vi "Begin.vi"(11 "Image Size":T1=enum."160x120") -> (0 "error out":errorcluster)   [LabVIEW 2012]
doc: "Called before other user functions, this VI is expected to open initial I/O refnums, load in file data, and do all program initialization. Notice that the <B>error out</B> terminal is simply used for data flow. Wiring it to other structures or subVIs ensures that this VI runs first."
uses:
  <vilib>/Rock Robotics/WPI/Camera/WPI_CameraImageSize.ctl
  <vilib>/Rock Robotics/WPI/Camera/WPI_CameraWhite Balance Values.ctl
  <vilib>/Rock Robotics/WPI/Camera/WPI_CameraExposure Values.ctl
  <vilib>/Rock Robotics/WPI/Camera/WPI_CameraFrameRate.ctl
  <vilib>/Rock Robotics/WPI/DriverStation/WPI_DriverStationRobotMode2.ctl
  <vilib>/Rock Robotics/WPI/Joystick/WPI_JoystickDeviceEnum.ctl
  <vilib>/Rock Robotics/SystemInterfaces/DIO/FPGA_DIOPWMChannel.ctl
  <vilib>/Rock Robotics/SystemInterfaces/Typedef/FPGA_TypedefDigitalModule.ctl
  <vilib>/Rock Robotics/SystemInterfaces/DIO/FPGA_DIORelayChannel.ctl
  <vilib>/Rock Robotics/WPI/Relay/WPI_RelayDirection.ctl
  <vilib>/Rock Robotics/WPI/AnalogChannel/WPI_AnalogChannelDevRef.ctl
  <vilib>/Rock Robotics/SystemInterfaces/Typedef/FPGA_TypedefAnalogModule.ctl
  <vilib>/Rock Robotics/SystemInterfaces/AI/FPGA_AIChannel.ctl
  <vilib>/Rock Robotics/SystemInterfaces/CounterEncoderSourceConvertion/FPGA_CounterEncoderSourceConvertionLVSourceType.ctl
  <vilib>/Rock Robotics/SystemInterfaces/DIO/FPGA_DIODigitalSourceChannel.ctl
  <vilib>/Rock Robotics/SystemInterfaces/AnalogTrigger/FPGA_AnalogTriggerIndex.ctl
  <vilib>/Rock Robotics/SystemInterfaces/AnalogTrigger/FPGA_AnalogTriggerOutType.ctl
  <vilib>/Rock Robotics/SystemInterfaces/AI/FPGA_AIGyroChannel.ctl
  <vilib>/Rock Robotics/SystemInterfaces/Typedef/FPGA_TypedefAnalogModuleForGyro.ctl
  <vilib>/Rock Robotics/SystemInterfaces/DIO/FPGA_DIOChannel.ctl
  <vilib>/Rock Robotics/WPI/Encoder/WPI_EncoderType.ctl
  Robot Global Data.vi
  <vilib>/Rock Robotics/WPI/RobotDrive/WPI_RobotDriveOpen2MotorWithJaguar.vi
  <vilib>/Rock Robotics/WPI/MotorControl/WPI_MotorControlOpen Victor.vi
  <vilib>/Rock Robotics/WPI/MotorControl/WPI_MotorControlOpen Jaguar.vi
  <vilib>/Rock Robotics/WPI/Counter/WPI_CounterOpen UpDown Mode.vi
  <vilib>/Rock Robotics/WPI/Counter/WPI_CounterDigitalInputToDigitalSource.vi
panel:
  out "error out 2":errorcluster
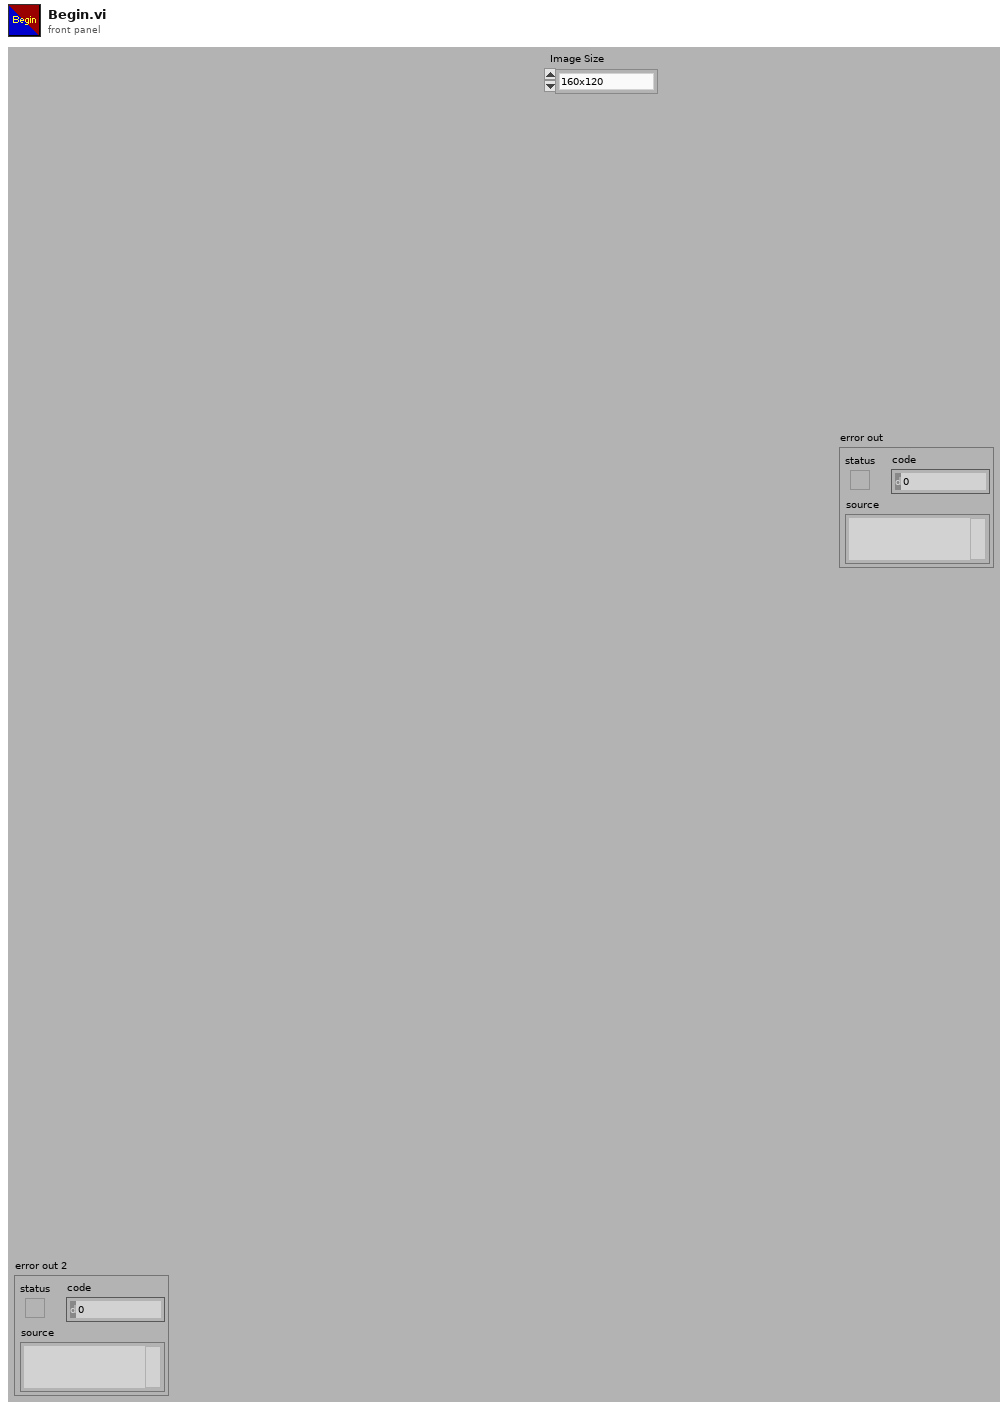
[diagram p1: front panel]
types:
  T1 = typedef "WPI_CameraImageSize.ctl" = enum16{"640x480", "320x240", "160x120"}
  T2 = typedef "WPI_RelayDirection.ctl" = enum16{"Both directions", "Forward only", "Reverse only"}
  T3 = typedef "FPGA_DIORelayChannel.ctl" = enum8{"Relay 1", "Relay 2", "Relay 3", "Relay 4", "Relay 5", "Relay 6", "Relay 7", "Relay 8", "Invalid"}
  T4 = typedef "FPGA_TypedefDigitalModule.ctl" = enum16{"Digital Module 1", "Digital Module 2"}
  T5 = typedef "FPGA_DIOPWMChannel.ctl" = enum8{"PWM 1", "PWM 2", "PWM 3", "PWM 4", "PWM 5", "PWM 6", "PWM 7", "PWM 8", "PWM 9", "PWM 10", "Invalid"}
  T6 = typedef "WPI_JoystickDeviceEnum.ctl" = enum16{"USB 1", "USB 2", "USB 3", "USB 4", "Kinect 1", "Kinect 2"}
  T7 = typedef "WPI_DriverStationRobotMode2.ctl" = enum16{"Autonomous Disabled", "Autonomous Enabled", "Teleop Disabled", "Teleop Enabled", "Timeout", "Finish", "Test Disabled", "Test Enabled"}
  T8 = typedef "WPI_CameraFrameRate.ctl" = u32
  T9 = typedef "WPI_CameraExposure Values.ctl" = enum16{"Auto", "Flicker-free 50 Hz", "Flicker-free 60 Hz", "Hold current"}
  T10 = typedef "WPI_CameraWhite Balance Values.ctl" = enum16{"Auto", "Fixed indoor", "Fixed outdoor 1", "Fixed outdoor 2", "Fixed fluorescent 1", "Fixed fluorescent 2", "Hold current"}
  T11 = enum16{"Rising Edge", "Falling Edge", "Raising & Falling Edge", "Disabled"}
  T12 = typedef "FPGA_CounterEncoderSourceConvertionLVSourceType.ctl" = cluster{"DevStatus":errorcluster, "AnalogTriggerMode?":bool, "DigitalMode":cluster{"Digital Module":T4, "DIO Channel":T13}, "AnalogTriggerMode":cluster{"AnalogTriggerIndex":T14, "OutputType":T15}}
  T13 = typedef "FPGA_DIODigitalSourceChannel.ctl" = enum8{"DIO 1", "DIO 2", "DIO 3", "DIO 4", "DIO 5", "DIO 6", "DIO 7", "DIO 8", "DIO 9", "DIO 10", "DIO 11", "DIO 12", "DIO 13", "DIO 14", "Disabled"}
  T14 = typedef "FPGA_AnalogTriggerIndex.ctl" = enum8{"Trig 0", "Trig 1", "Trig 2", "Trig 3", "Trig 4", "Trig 5", "Trig 6", "Trig 7", "Invalid"}
  T15 = typedef "FPGA_AnalogTriggerOutType.ctl" = enum16{"InWindow", "TriggerState", "Rising", "Falling"}
  T16 = typedef "WPI_AnalogChannelDevRef.ctl" = cluster{"DevStatus":errorcluster, "Analog Module":T17, "Analog Channel":T18}
  T17 = typedef "FPGA_TypedefAnalogModule.ctl" = enum16{"Analog Module 1", "Analog Module 2"}
  T18 = typedef "FPGA_AIChannel.ctl" = enum8{"AI 1", "AI 2", "AI 3", "AI 4", "AI 5", "AI 6", "AI 7", "AI 8", "Invalid"}
  T19 = typedef "FPGA_AnalogTriggerDevRef.ctl" = cluster{"DevStatus":errorcluster, "AnalogTriggerIndex":T14}
  T20 = typedef "WPI_CounterDevRef.ctl" = cluster{"DevStatus":errorcluster, "CntIndex":T21}
  T21 = typedef "FPGA_CounterCtrSystemIndex.ctl" = enum8{"Ctr 0", "Ctr 1", "Ctr 2", "Ctr 3", "Ctr 4", "Ctr 5", "Ctr 6", "Ctr 7", "Invalid"}
  T22 = typedef "WPI_MotorControlDeviceRef.ctl" = cluster{"DeviceStatus":errorcluster, "Type":enum16{"PWM", "CAN"}, "PWM":cluster{"Digital Module":T4, "PWM Channel":T5, "DeadBand":T23}, "CAN":cluster{"Device Number":u8, "Control Mode":T24, "Semaphore":T25, "Max Vout":dbl}, "Invert":bool, "TransformRef":T26, "InvTransformRef":T26}
  T23 = typedef "WPI_PWMDeadband.ctl" = cluster{"Name":string, "maxPositivePwm":i32, "minPositivePwm":i32, "centerPwm":i32, "maxNegativePwm":i32, "minNegativePwm":i32, "angularRange":u16}
  T24 = typedef "WPI_CANJaguar_ControlMode.ctl" = enum8{"Percent VBus", "Current", "Speed", "Position", "Voltage"}
  T25 = typedef "Semaphore RefNum" = refnum<k1>
  T26 = typedef "WPI_PWMTransform_ConPane.ctl" = refnum<vi>
  T27 = typedef "WPI_CameraDevRef.ctl" = cluster{"Camera Address":string, "CameraStatus":errorcluster, "Acquire Image Notifier":refnum<notifier>}
  T28 = typedef "WPI_JoystickDevRef.ctl" = cluster{"Device":T6}
  T29 = typedef "WPI_RelayDevRef.ctl" = cluster{"DevStatus":errorcluster, "Relay Channel":T3, "Digital Module":T4, "Relay Direction":T2}
  T30 = typedef "WPI_RobotDriveDevRef.ctl" = cluster{"DevStatus":errorcluster, "Motors[]":T22[], "Square Inputs":bool, "Max Output":dbl, "Isochronous":bool}
  T31 = typedef "FPGA_AIGyroChannel.ctl" = enum8{"AI 1", "AI 2", "Invalid"}
  T32 = typedef "FPGA_TypedefAnalogModuleForGyro.ctl" = enum16{"Analog Module 1"}
  T33 = typedef "WPI_GyroDevRef.ctl" = cluster{"DevStatus":errorcluster, "Analog Module":T17, "Analog Channel":T18, "Offset":dbl, "Gain (VoltsPerDegree/Second)":dbl}
  T34 = typedef "WPI_EncoderType.ctl" = enum16{"1x", "2x", "4x"}
  T35 = typedef "FPGA_DIOChannel.ctl" = enum8{"DIO 1", "DIO 2", "DIO 3", "DIO 4", "DIO 5", "DIO 6", "DIO 7", "DIO 8", "DIO 9", "DIO 10", "DIO 11", "DIO 12", "DIO 13", "DIO 14", "Invalid"}
  T36 = typedef "WPI_DigitalInputDevRef.ctl" = cluster{"DevStatus":errorcluster, "DIO Channel":T35, "Digital Module":T4}
  T37 = typedef "WPI_EncoderDevRef.ctl" = cluster{"DevStatus":errorcluster, "EncoderIndex":T38, "CounterIndex":T21, "DistancePerCount":dbl, "Decoding Type":T34}
  T38 = typedef "FPGA_EncoderIdx.ctl" = enum8{"Enc 0", "Enc 1", "Enc 2", "Enc 3", "Invalid"}
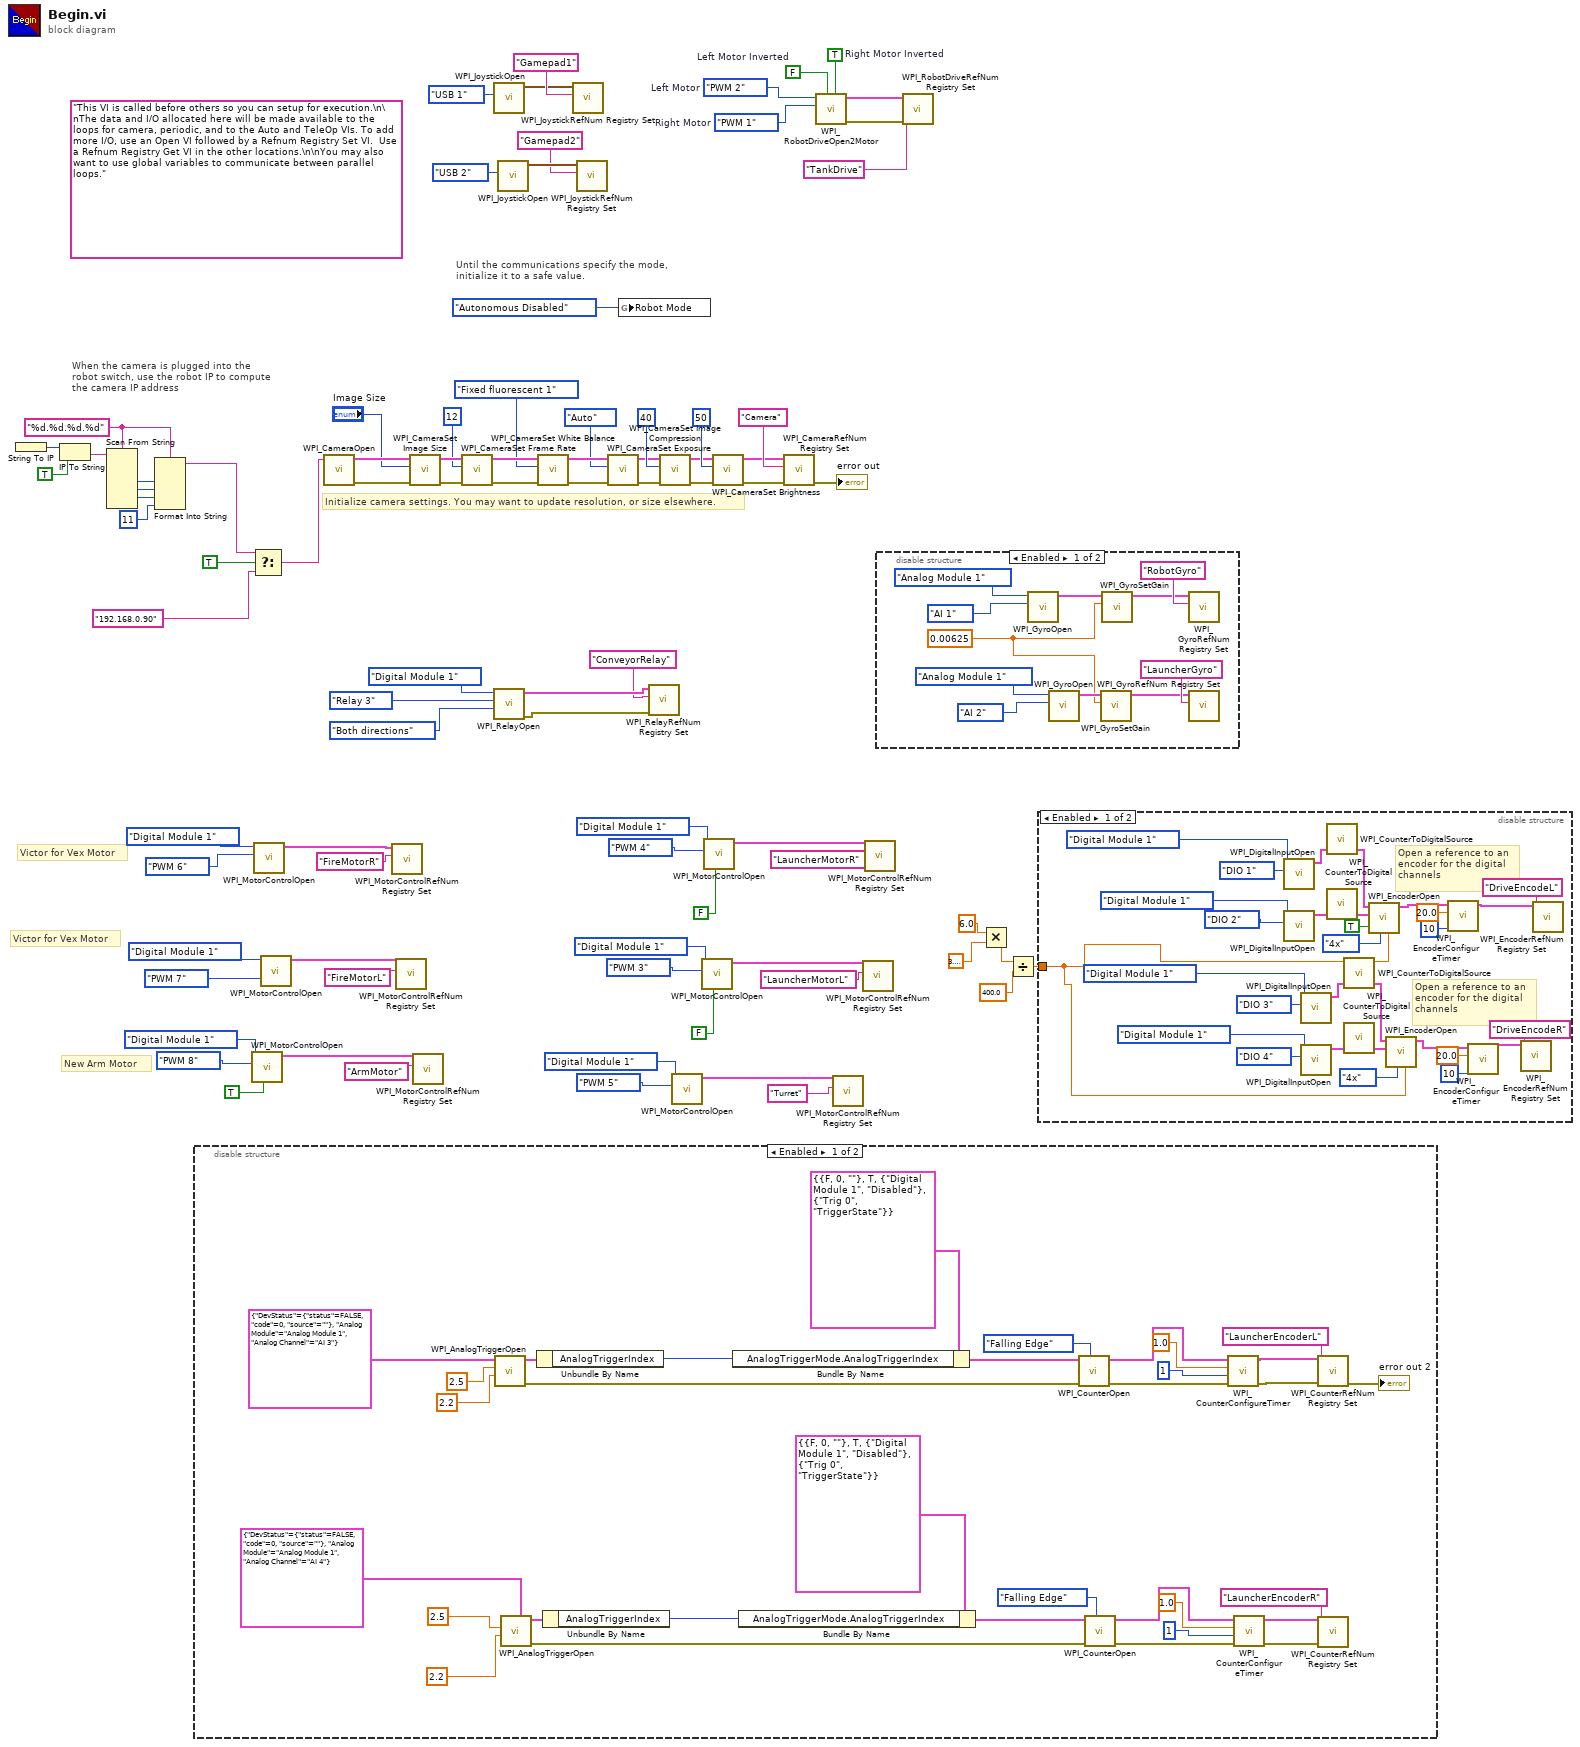
[diagram p0: block diagram]
diagram:
  w43 = FPGA_DIOPWMChannel."PWM 1"  # Right Motor
  w44 = FPGA_DIOPWMChannel."PWM 2"  # Left Motor
  w45 = TRUE  # Right Motor Inverted
  w46 = FALSE  # Left Motor Inverted
  w58 = "%d.%d.%d.%d" ("format string")
  (unwired) "This VI is called before others so you can setup for execution.\n\nThe data and I/O allocated here will be made available to the loops for camera, periodic, and to the Auto and TeleOp VIs. To add more I/O, use an Open VI followed by a Refnum Registry Set VI.  Use a Refnum Registry Get VI in the other locations.\n\nYou may also want to use global variables to communicate between parallel loops."
  # "New Arm Motor"
  # "Victor for Vex Motor"
  # "Victor for Vex Motor"
  # "Until the communications specify the mode,\ninitialize it to a safe value."
  # "When the camera is plugged into the\nrobot switch, use the robot IP to compute\nthe camera IP address"
  # "Initialize camera settings. You may want to update resolution, or size elsewhere."
  n1 = String To IP() -> (0:w65:u32)  [unwired: 1 in]
  n2 = IP To String(1:TRUE ("dot notation? (F)"), 2:w65) -> (0:w63:string)
  n3 = Scan From String(format string=w58, input string=w63) -> (output 1=w62:i32, output 2=w61:i32, output 3=w60:i32)  [unwired: 7 in, 3 out]
  n4 = Format Into String(format string=w58, w62, w61, w60, 11 ("Compression")) -> (resulting string=w28:string)  [unwired: 2 in, 1 out]
  n5 = disable-structure shown="Enabled" {
    frame Enabled {
      n6 = call <vilib>:"WPI_AnalogTriggerOpen.vi"("LowerLimit (v)"=2.2, "UpperLimit (v)"=2.5, "AnalogTriggerSource"=T16 {"DevStatus"={"status"=FALSE, "code"=0, "source"=""}, "Analog Module"=enum."Analog Module 1", "Analog Channel"=enum."AI 3"}) -> ("error out"=w118:errorcluster, "AnalogTriggerDevRef"=w111:T19)  [unwired: 7 in]
      n7 = call <vilib>:"WPI_AnalogTriggerOpen.vi"("LowerLimit (v)"=2.2 ("LowerLimit (v) 2"), "UpperLimit (v)"=2.5 ("UpperLimit (v) 2"), "AnalogTriggerSource"=T16 {"DevStatus"={"status"=FALSE, "code"=0, "source"=""}, "Analog Module"=enum."Analog Module 1", "Analog Channel"=enum."AI 4"} ("AnalogTriggerSource 2")) -> ("error out"=w105:errorcluster, "AnalogTriggerDevRef"=w98:T19)  [unwired: 7 in]
      n8 = Unbundle By Name(w111) -> ("AnalogTriggerIndex"=w110:T14)
      n9 = Unbundle By Name(w98) -> ("AnalogTriggerIndex"=w97:T14)
      n10 = Bundle By Name(cluster=T12 {"DevStatus"={"status"=FALSE, "code"=0, "source"=""}, "AnalogTriggerMode?"=TRUE, "DigitalMode"={"Digital Module"=enum."Digital Module 1", "DIO Channel"=enum."Disabled"}, "AnalogTriggerMode"={"AnalogTriggerIndex"=enum."Trig 0", "OutputType"=enum."TriggerState"}} ("Source"), "AnalogTriggerMode.AnalogTriggerIndex"=w110) -> (w108:T12)
      n11 = Bundle By Name(cluster=T12 {"DevStatus"={"status"=FALSE, "code"=0, "source"=""}, "AnalogTriggerMode?"=TRUE, "DigitalMode"={"Digital Module"=enum."Digital Module 1", "DIO Channel"=enum."Disabled"}, "AnalogTriggerMode"={"AnalogTriggerIndex"=enum."Trig 0", "OutputType"=enum."TriggerState"}} ("Source 2"), "AnalogTriggerMode.AnalogTriggerIndex"=w97) -> (w95:T12)
      n12 = call-poly <vilib>:"WPI_CounterOpen.vi"("UpEdge"=T11."Falling Edge" ("UpEdge 1"), "error in (no error)"=w118, "Up Source"=w108) -> ("error out"=w114:errorcluster, "CounterDevRef"=w115:T20)  [unwired: 7 in]
      n13 = call-poly <vilib>:"WPI_CounterOpen.vi"("UpEdge"=T11."Falling Edge" ("UpEdge 2"), "error in (no error)"=w105, "Up Source"=w95) -> ("error out"=w101:errorcluster, "CounterDevRef"=w102:T20)  [unwired: 7 in]
      n14 = call <vilib>:"WPI_CounterConfigureTimer.vi"("error in (no error)"=w114, "Number Samples to Average"=u8 1, "MaxPeriod (sec)"=1.0, "CounterDevRef in"=w115) -> ("error out"=w88:errorcluster, "CounterDevRef out"=w89:T20)  [unwired: 6 in]
      n15 = call <vilib>:"WPI_CounterConfigureTimer.vi"("error in (no error)"=w101, "Number Samples to Average"=u8 1, "MaxPeriod (sec)"=1.0, "CounterDevRef in"=w102) -> ("error out"=w92:errorcluster, "CounterDevRef out"=w93:T20)  [unwired: 6 in]
      n16 = call <vilib>:"WPI_CounterRefNum Registry Set.vi"("error in (no error)"=w88, "refnum name"="LauncherEncoderL", "CounterDevRef"=w89) -> ("error out"=→"error out 2":errorcluster)  [unwired: 7 in, 1 out]
      n17 = call <vilib>:"WPI_CounterRefNum Registry Set.vi"("error in (no error)"=w92, "refnum name"="LauncherEncoderR", "CounterDevRef"=w93) -> ()  [unwired: 7 in, 2 out]
    }
    frame Disabled {
    }
  }
  n18 = call-poly <vilib>:"WPI_MotorControlOpen.vi"("Invert"=TRUE, "PWM Channel"=FPGA_DIOPWMChannel."PWM 8", "Digital Module (Module 1)"=FPGA_TypedefDigitalModule."Digital Module 1") -> ("MotorControlDeviceRef"=w42:T22)  [unwired: 7 in, 1 out]
  n19 = Select(t=w28, s=TRUE, f="192.168.0.90") -> (s? t:f=w27:string)
  n20 = call-poly <vilib>:"WPI_MotorControlOpen.vi"("PWM Channel"=FPGA_DIOPWMChannel."PWM 6", "Digital Module (Module 1)"=FPGA_TypedefDigitalModule."Digital Module 1") -> ("MotorControlDeviceRef"=w40:T22)  [unwired: 8 in, 1 out]
  n21 = call-poly <vilib>:"WPI_MotorControlOpen.vi"("PWM Channel"=FPGA_DIOPWMChannel."PWM 7", "Digital Module (Module 1)"=FPGA_TypedefDigitalModule."Digital Module 1") -> ("MotorControlDeviceRef"=w41:T22)  [unwired: 8 in, 1 out]
  n22 = call <vilib>:"WPI_CameraOpen.vi"("Camera Address"=w27) -> ("error out"=w77:errorcluster, "CameraDevRef"=w78:T27)  [unwired: 1 in, 8 out]
  n23 = call <vilib>:"WPI_MotorControlRefNum Registry Set.vi"("refnum name"="FireMotorR", "MotorControlDevRef"=w40) -> ()  [unwired: 8 in, 2 out]
  n24 = call <vilib>:"WPI_MotorControlRefNum Registry Set.vi"("refnum name"="FireMotorL", "MotorControlDevRef"=w41) -> ()  [unwired: 8 in, 2 out]
  n25 = call <vilib>:"WPI_CameraSet Image Size.vi"("error in (no error)"=w77, "Image Size"="Image Size", "CameraDevRef"=w78) -> ("error out"=w76:errorcluster, "CameraDevRef Out"=w79:T27)  [unwired: 7 out]
  n26 = call <vilib>:"WPI_MotorControlRefNum Registry Set.vi"("refnum name"="ArmMotor", "MotorControlDevRef"=w42) -> ()  [unwired: 8 in, 2 out]
  n27 = call <vilib>:"WPI_CameraSet Frame Rate.vi"("error in (no error)"=w76, "Frame Rate (fps)"=T8 12, "CameraDevRef"=w79) -> ("error out"=w75:errorcluster, "CameraDevRef Out"=w81:T27)  [unwired: 7 out]
  n28 = call <vilib>:"WPI_JoystickOpen.vi"("JoystickDevice"=WPI_JoystickDeviceEnum."USB 1") -> ("JoystickDevRef"=w55:T28)  [unwired: 10 in]
  n29 = call <vilib>:"WPI_RelayOpen.vi"("Relay Direction"=WPI_RelayDirection."Both directions", "Relay Channel"=FPGA_DIORelayChannel."Relay 3", "Digital Module (Module 1)"=FPGA_TypedefDigitalModule."Digital Module 1") -> ("error out"=w11:errorcluster, "RelayDevRef"=w12:T29)  [unwired: 7 in]
  n30 = call <vilib>:"WPI_JoystickOpen.vi"("JoystickDevice"=WPI_JoystickDeviceEnum."USB 2") -> ("JoystickDevRef"=w51:T28)  [unwired: 10 in]
  n31 = call <vilib>:"WPI_CameraSet White Balance.vi"("error in (no error)"=w75, "White Balance"=WPI_CameraWhite_Balance_Values."Fixed fluorescent 1", "CameraDevRef"=w81) -> ("error out"=w74:errorcluster, "CameraDevRef Out"=w80:T27)  [unwired: 7 out]
  n32 = call <vilib>:"WPI_JoystickRefNum Registry Set.vi"("refnum name"="Gamepad1", "JoystickDevRef"=w55) -> ()  [unwired: 8 in, 2 out]
  n33 = call <vilib>:"WPI_JoystickRefNum Registry Set.vi"("refnum name"="Gamepad2", "JoystickDevRef"=w51) -> ()  [unwired: 8 in, 2 out]
  n34 = call <vilib>:"WPI_CameraSet Exposure.vi"("error in (no error)"=w74, "Exposure"=WPI_CameraExposure_Values."Auto", "CameraDevRef"=w80) -> ("error out"=w73:errorcluster, "CameraDevRef Out"=w83:T27)  [unwired: 7 out]
  n35 = global write "Robot Global Data.vi" "Robot Mode"(WPI_DriverStationRobotMode2."Autonomous Disabled" ("Robot Mode")) -> ()
  n36 = call <vilib>:"WPI_RelayRefNum Registry Set.vi"("error in (no error)"=w11, "refnum name"="ConveyorRelay", "RelayDevRef"=w12) -> ()  [unwired: 7 in, 2 out]
  n37 = call <vilib>:"WPI_CameraSet Image Compression.vi"("error in (no error)"=w73, "Compression"=40, "CameraDevRef"=w83) -> ("error out"=w72:errorcluster, "CameraDevRef Out"=w82:T27)  [unwired: 7 out]
  n38 = call-poly <vilib>:"WPI_MotorControlOpen.vi"("PWM Channel"=FPGA_DIOPWMChannel."PWM 5", "Digital Module (Module 1)"=FPGA_TypedefDigitalModule."Digital Module 1") -> ("MotorControlDeviceRef"=w16:T22)  [unwired: 8 in, 1 out]
  n39 = call-poly <vilib>:"WPI_MotorControlOpen.vi"("Invert"=FALSE, "PWM Channel"=FPGA_DIOPWMChannel."PWM 3", "Digital Module (Module 1)"=FPGA_TypedefDigitalModule."Digital Module 1") -> ("MotorControlDeviceRef"=w26:T22)  [unwired: 7 in, 1 out]
  n40 = call-poly <vilib>:"WPI_MotorControlOpen.vi"("Invert"=FALSE, "PWM Channel"=FPGA_DIOPWMChannel."PWM 4", "Digital Module (Module 1)"=FPGA_TypedefDigitalModule."Digital Module 1") -> ("MotorControlDeviceRef"=w21:T22)  [unwired: 7 in, 1 out]
  n41 = call <vilib>:"WPI_CameraSet Brightness.vi"("error in (no error)"=w72, "Brightness"=50, "CameraDevRef"=w82) -> ("error out"=w70:errorcluster, "CameraDevRef Out"=w71:T27)  [unwired: 7 out]
  n42 = call <vilib>:"WPI_CameraRefNum Registry Set.vi"("error in (no error)"=w70, "refnum name"="Camera", "CameraDevRef"=w71) -> ("error out"=→"error out":errorcluster)  [unwired: 8 out]
  n43 = call-poly <vilib>:"WPI_RobotDriveOpen2Motor.vi"("Right Motor Inverted"=w45, "Left Motor Inverted"=w46, "Right Motor"=w43, "Left Motor"=w44) -> ("error out"=w47:errorcluster, "RobotDriveDevRef"=w49:T30)  [unwired: 6 in]
  n44 = call <vilib>:"WPI_MotorControlRefNum Registry Set.vi"("refnum name"="Turret", "MotorControlDevRef"=w16) -> ()  [unwired: 8 in, 2 out]
  n45 = call <vilib>:"WPI_MotorControlRefNum Registry Set.vi"("refnum name"="LauncherMotorL", "MotorControlDevRef"=w26) -> ()  [unwired: 8 in, 2 out]
  n46 = call <vilib>:"WPI_MotorControlRefNum Registry Set.vi"("refnum name"="LauncherMotorR", "MotorControlDevRef"=w21) -> ()  [unwired: 8 in, 2 out]
  n47 = disable-structure shown="Enabled" {
    frame Enabled {
      w120 = 0.00625
      n48 = call <vilib>:"WPI_GyroOpen.vi"("Analog Channel"=FPGA_AIGyroChannel."AI 1", "Analog Module (Module 1)"=FPGA_TypedefAnalogModuleForGyro."Analog Module 1") -> ("GyroDevRef"=w124:T33)  [unwired: 7 in, 2 out]
      n49 = call <vilib>:"WPI_GyroOpen.vi"("Analog Channel"=FPGA_AIGyroChannel."AI 2", "Analog Module (Module 1)"=FPGA_TypedefAnalogModuleForGyro."Analog Module 1") -> ("GyroDevRef"=w122:T33)  [unwired: 7 in, 2 out]
      n50 = call <vilib>:"WPI_GyroSetGain.vi"("Gain (VoltsPerDegree/Second)"=w120, "GyroDevRef"=w122) -> ("GyroDevRef"=w121:T33)  [unwired: 8 in, 1 out]
      n51 = call <vilib>:"WPI_GyroSetGain.vi"("Gain (VoltsPerDegree/Second)"=w120, "GyroDevRef"=w124) -> ("GyroDevRef"=w123:T33)  [unwired: 8 in, 1 out]
      n52 = call <vilib>:"WPI_GyroRefNum Registry Set.vi"("refnum name"="RobotGyro", "GyroDevRef"=w123) -> ()  [unwired: 8 in, 2 out]
      n53 = call <vilib>:"WPI_GyroRefNum Registry Set.vi"("refnum name"="LauncherGyro", "GyroDevRef"=w121) -> ()  [unwired: 8 in, 2 out]
    }
    frame Disabled {
    }
  }
  n54 = call <vilib>:"WPI_RobotDriveRefNum Registry Set.vi"("error in (no error)"=w47, "refnum name"="TankDrive", "RobotDriveDevRef"=w49) -> ()  [unwired: 7 in, 2 out]
  n55 = Multiply(x=6.0, y=3.141592653589793) -> (x*y=w3:dbl)
  n56 = Divide(x=w3, y=400.0) -> (x/y=w1:dbl)
  n57 = disable-structure shown="Enabled" {
    disable-tunnel: w1 -> [w132 _]
    frame Enabled {
      # "Open a reference to an\nencoder for the digital \nchannels"
      # "Open a reference to an\nencoder for the digital \nchannels"
      n58 = call <vilib>:"WPI_DigitalInputOpen.vi"("DIO Channel"=FPGA_DIOChannel."DIO 1", "Digital Module (Module 1)"=FPGA_TypedefDigitalModule."Digital Module 1") -> ("DigitalInputDevRef"=w158:T36)  [unwired: 1 in, 8 out]
      n59 = call <vilib>:"WPI_DigitalInputOpen.vi"("DIO Channel"=FPGA_DIOChannel."DIO 2", "Digital Module (Module 1)"=FPGA_TypedefDigitalModule."Digital Module 1") -> ("DigitalInputDevRef"=w159:T36)  [unwired: 1 in, 8 out]
      n60 = call <vilib>:"WPI_DigitalInputOpen.vi"("DIO Channel"=FPGA_DIOChannel."DIO 3", "Digital Module (Module 1)"=FPGA_TypedefDigitalModule."Digital Module 1") -> ("DigitalInputDevRef"=w148:T36)  [unwired: 1 in, 8 out]
      n61 = call <vilib>:"WPI_DigitalInputOpen.vi"("DIO Channel"=FPGA_DIOChannel."DIO 4", "Digital Module (Module 1)"=FPGA_TypedefDigitalModule."Digital Module 1") -> ("DigitalInputDevRef"=w149:T36)  [unwired: 1 in, 8 out]
      n62 = call-poly <vilib>:"WPI_CounterToDigitalSource.vi"("DigitalInputDevRef"=w158) -> ("Digital Source"=w157:T12)  [unwired: 6 out]
      n63 = call-poly <vilib>:"WPI_CounterToDigitalSource.vi"("DigitalInputDevRef"=w159) -> ("Digital Source"=w160:T12)  [unwired: 6 out]
      n64 = call-poly <vilib>:"WPI_CounterToDigitalSource.vi"("DigitalInputDevRef"=w148) -> ("Digital Source"=w147:T12)  [unwired: 6 out]
      n65 = call-poly <vilib>:"WPI_CounterToDigitalSource.vi"("DigitalInputDevRef"=w149) -> ("Digital Source"=w150:T12)  [unwired: 6 out]
      n66 = call <vilib>:"WPI_EncoderOpen.vi"("DistancePerCount"=w132, "Decoding Type"=WPI_EncoderType."4x", "Invert Direction (False)"=TRUE, "BSource"=w160, "ASource"=w157) -> ("EncoderDevRef"=w154:T37)  [unwired: 3 in, 3 out]
      n67 = call <vilib>:"WPI_EncoderOpen.vi"("DistancePerCount"=w132, "Decoding Type"=WPI_EncoderType."4x", "BSource"=w150, "ASource"=w147) -> ("EncoderDevRef"=w146:T37)  [unwired: 4 in, 3 out]
      n68 = call <vilib>:"WPI_EncoderConfigureTimer.vi"("Number Samples to Average"=u8 10, "Minimum Rate"=20.0, "EncoderDevRef"=w154) -> ("EncoderDevRef"=w151:T37)  [unwired: 1 in, 7 out]
      n69 = call <vilib>:"WPI_EncoderConfigureTimer.vi"("Number Samples to Average"=u8 10, "Minimum Rate"=20.0, "EncoderDevRef"=w146) -> ("EncoderDevRef"=w143:T37)  [unwired: 1 in, 7 out]
      n70 = call <vilib>:"WPI_EncoderRefNum Registry Set.vi"("refnum name"="DriveEncodeR", "EncoderDevRef"=w143) -> ()  [unwired: 8 in, 2 out]
      n71 = call <vilib>:"WPI_EncoderRefNum Registry Set.vi"("refnum name"="DriveEncodeL", "EncoderDevRef"=w151) -> ()  [unwired: 8 in, 2 out]
    }
    frame Disabled {
    }
  }
